vi "Read ADXL345.vi"(10 "Private Data In":T1) -> (0 "Z (g)":fxp<+/-,32,10>, 1 "Y (g)":fxp<+/-,32,10>, 2 "X (g)":fxp<+/-,32,10>, 3 "Private Data Out":T1)   [LabVIEW 2014]
uses:
  <vilib>/IEDriver/SPIandI2C/FPGA/Type Def/Private Data (SPI).ctl
  <vilib>/IEDriver/SPIandI2C/FPGA/Library/IP SPI&I2C.lvlib
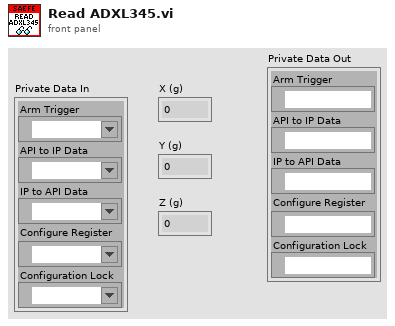
[diagram p1: front panel]
types:
  T1 = typedef "IP SPI&I2C.lvlib/Private Data (SPI).ctl" = cluster{"Arm Trigger":refnum<k21>, "API to IP Data":refnum<k21>, "IP to API Data":refnum<k21>, "Configure Register":refnum<k21>, "Configuration Lock":refnum<k21>}
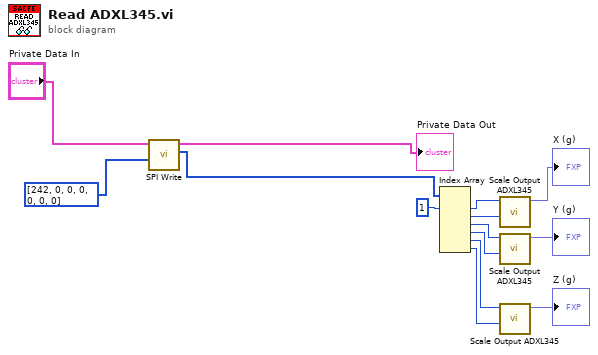
[diagram p0: block diagram]
diagram:
  n1 = call "SPI Write.vi"("Write Data"=u8[] [242, 0, 0, 0, 0, 0, 0], "Private Data In"="Private Data In") -> ("Read Out"=w4:u8[], "Private Data Out"=→"Private Data Out":T1)  [unwired: 8 in]
  n2 = Index Array(array=w4, index #1=1 ("index")) -> (element #1=w6:u8, element #2=w7:u8, element #3=w8:u8, element #4=w9:u8, element #5=w10:u8, element #6=w11:u8)  [unwired: 5 in]
  n3 = call "Scale Output ADXL345.vi"("Byte1"=w7, "Byte0"=w6) -> ("G's"=→"X (g)":fxp<+/-,32,10>)  [unwired: 9 in]
  n4 = call "Scale Output ADXL345.vi"("Byte1"=w9, "Byte0"=w8) -> ("G's"=→"Y (g)":fxp<+/-,32,10>)  [unwired: 9 in]
  n5 = call "Scale Output ADXL345.vi"("Byte1"=w11, "Byte0"=w10) -> ("G's"=→"Z (g)":fxp<+/-,32,10>)  [unwired: 9 in]
